vi "Export - Main.vi"(8 "error in (no error)":errorcluster, 11 "Device Item Ref in":T10 format="%.0x") -> (0 "error out":errorcluster, 3 "Import/Export Data":T1 {"Tx Packets"."Tx Packet Data"."Endianness" items=["big-endian"=0, "little-endian"=2]; "Rx Packets"."Rx Packet Data"."Endianness" items=["big-endian"=0, "little-endian"=2]})   [LabVIEW 2016, in "UDP-Custom-Device System Explorer.lvlib"]
uses:
  UDP-Custom-Device System Explorer.lvlib
  <vilib>/NI Veristand/Custom Device API/Custom Device Item Ref.ctl
  Types/XML - New/ImpExp - Data.ctl
  Types/XML - New/ImpExp - Main Data.ctl
  <vilib>/NI Veristand/Custom Device API/Custom Device Item Info.ctl
  Types/XML - New/ImpExp - Rx Packets Data.ctl
  Types/XML - New/ImpExp - Rx Packet Data.ctl
  Shared/Types/Shared - Channel Data Type.ctl
  Shared/Types/Shared - Buffered.PacketInfo.ctl
  Types/XML - New/ImpExp - Tx Packets Data.ctl
  Types/XML - New/ImpExp - Tx Packet Data.ctl
  Property Accessors/Main Accessors.lvlib
  <vilib>/NI VeriStand/Custom Device API/Custom Device API.lvlib
  Shared/UDP-Custom-Device Shared.lvlib
  <vilib>/NI VeriStand/Custom Device Tools/Custom Device Utility Library/Custom Device Utility Library.lvlib
panel:
  out "Controller Path":string
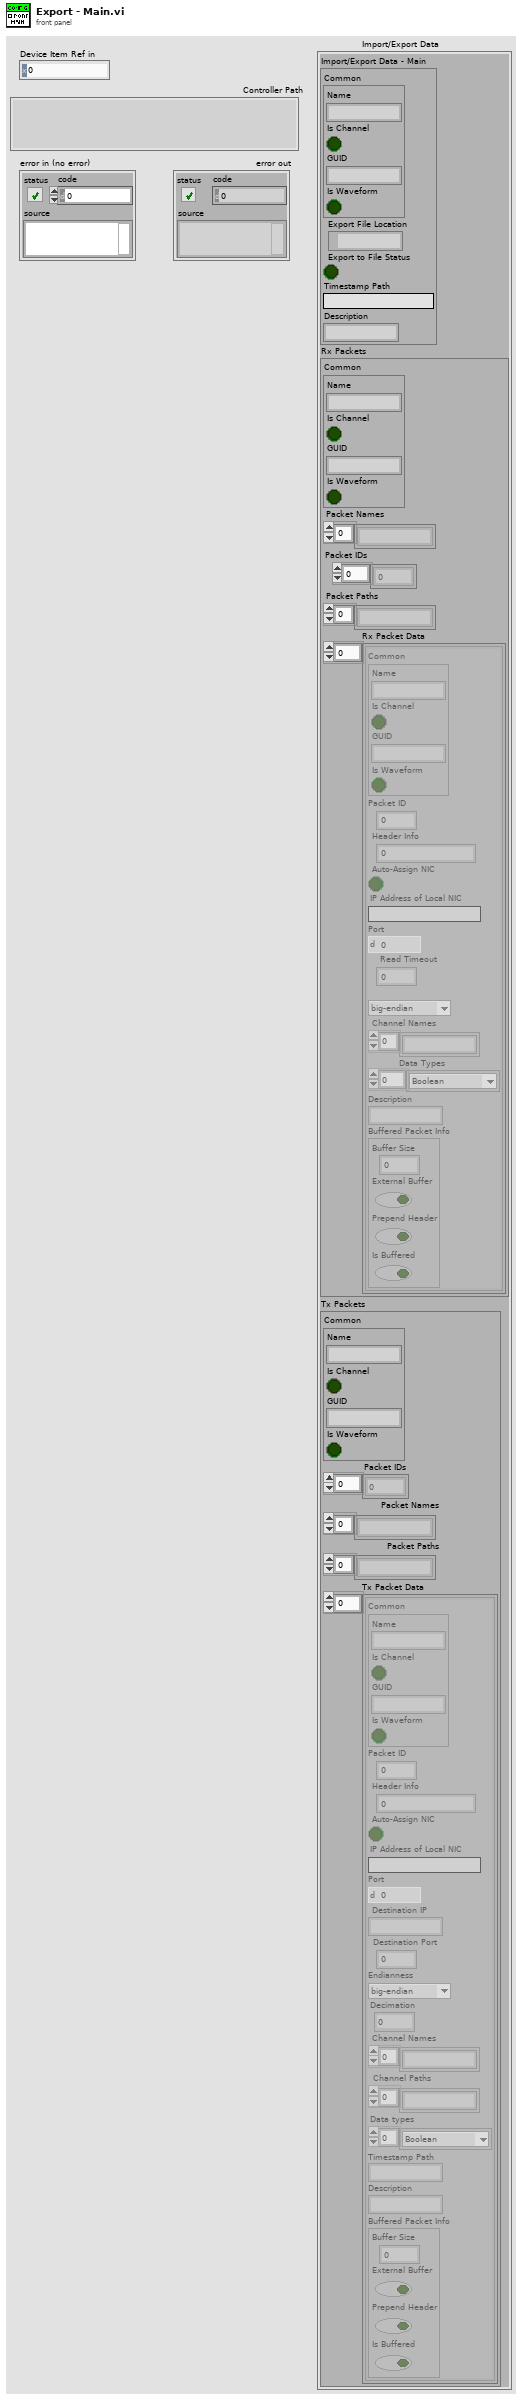
[diagram p1: front panel]
types:
  T1 = typedef "UDP-Custom-Device System Explorer.lvlib/ImpExp - Data.ctl" = cluster{"Import/Export Data - Main":T2, "Rx Packets":T4, "Tx Packets":T8}
  T2 = typedef "UDP-Custom-Device System Explorer.lvlib/ImpExp - Main Data.ctl" = cluster{"Common":T3, "Export File Location":path, "Export to File Status":bool, "Timestamp Path":string, "Description":string}
  T3 = typedef "Custom Device API.lvlib/Custom Device Item Info.ctl" = cluster{"Name":string, "Is Channel":bool, "GUID":string, "Is Waveform":bool}
  T4 = typedef "UDP-Custom-Device System Explorer.lvlib/ImpExp - Rx Packets Data.ctl" = cluster{"Common":T3, "Packet Names":string[], "Packet IDs":i32[], "Packet Paths":string[], "Rx Packet Data":T5[]}
  T5 = typedef "UDP-Custom-Device System Explorer.lvlib/ImpExp - Rx Packet Data.ctl" = cluster{"Common":T3, "Packet ID":i32, "Header Info":u32, "Auto-Assign NIC":bool, "IP Address of Local NIC":string, "Port":u16, "Read Timeout":i32, "Endianness":u16, "Channel Names":string[], "Data Types":T6[], "Description":string, "Buffered Packet Info":T7}
  T6 = typedef "UDP-Custom-Device Shared.lvlib/Shared - Channel Data Type.ctl" = enum16{"Boolean", "Single", "Double", "I8", "I16", "I32", "I64", "U8", "U16", "U32", "U64"}
  T7 = typedef "UDP-Custom-Device Shared.lvlib/Shared - Buffered.PacketInfo.ctl" = cluster{"Buffer Size":i32, "External Buffer":bool, "Prepend Header":bool, "Is Buffered":bool}
  T8 = typedef "UDP-Custom-Device System Explorer.lvlib/ImpExp - Tx Packets Data.ctl" = cluster{"Common":T3, "Packet IDs":i32[], "Packet Names":string[], "Packet Paths":string[], "Tx Packet Data":T9[]}
  T9 = typedef "UDP-Custom-Device System Explorer.lvlib/ImpExp - Tx Packet Data.ctl" = cluster{"Common":T3, "Packet ID":i32, "Header Info":u32, "Auto-Assign NIC":bool, "IP Address of Local NIC":string, "Port":u16, "Destination IP":string, "Destination Port":u16, "Endianness":u16, "Decimation":u16, "Channel Names":string[], "Channel Paths":string[], "Data types":T6[], "Timestamp Path":string, "Description":string, "Buffered Packet Info":T7}
  T10 = typedef "Custom Device API.lvlib/Custom Device Item Ref.ctl" = u64
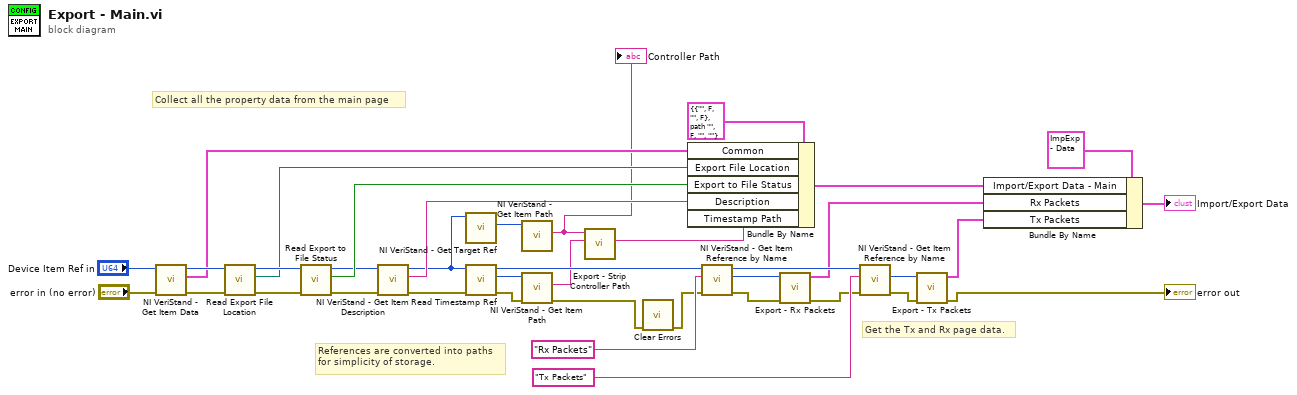
[diagram p0: block diagram]
diagram:
  # "References are converted into paths\nfor simplicity of storage."
  # "Get the Tx and Rx page data."
  # "Collect all the property data from the main page"
  n1 = call <vilib>:"NI VeriStand - Get Item Data.vi"("error in (no error)"="error in (no error)", "Item Ref in"="Device Item Ref in") -> ("error out"=w31:errorcluster, "Item Info"=w28:T3, "Item Ref out"=w33:T10)  [unwired: 6 in, 1 out]
  n2 = call "Read Export File Location.vi"("error in (no error)"=w31, "Node Ptr"=w33) -> ("error out"=w38:errorcluster, "Export File Location"=w27:path, "Node Ptr out"=w37:T10)  [unwired: 7 in]
  n3 = call "Read Export to File Status.vi"("error in (no error)"=w38, "Node Ptr"=w37) -> ("error out"=w9:errorcluster, "Export to File Status"=w26:bool, "Node Ptr out"=w6:T10)  [unwired: 7 in]
  n4 = call <vilib>:"NI VeriStand - Get Item Description.vi"("error in (no error)"=w9, "Item Ref in"=w6) -> ("error out"=w8:errorcluster, "Description"=w5:string, "Item Ref out"=w4:T10)  [unwired: 6 in, 1 out]
  n5 = call <vilib>:"NI VeriStand - Get Target Ref.vi"("Item Ref in"=w4) -> ("Target Ref"=w7:T10)  [unwired: 7 in, 3 out]
  n6 = call "Read Timestamp Ref.vi"("error in (no error)"=w8, "Node Ptr"=w4) -> ("error out"=w35:errorcluster, "Timestamp Ref"=w36:T10, "Node Ptr out"=w24:T10)  [unwired: 7 in]
  n7 = call <vilib>:"NI VeriStand - Get Item Path.vi"("Item Ref in"=w7) -> ("Path"=w1:string)  [unwired: 7 in, 3 out]
  "Controller Path" <- w1
  n8 = call <vilib>:"NI VeriStand - Get Item Path.vi"("error in (no error)"=w35, "Item Ref in"=w36) -> ("error out"=w11:errorcluster, "Path"=w3:string)  [unwired: 6 in, 2 out]
  n9 = call "Export - Strip Controller Path.vi"("Channel Path"=w3, "Controller Path"=w1) -> ("Stripped Path"=w2:string)  [unwired: 8 in, 1 out]
  n10 = call <vilib>:"Clear Errors.vi"("error in (no error)"=w11) -> ("error out"=w10:errorcluster)  [unwired: 5 in, 1 out]
  n11 = Bundle By Name(cluster=T2 {"Common"={"Name"="", "Is Channel"=FALSE, "GUID"="", "Is Waveform"=FALSE}, "Export File Location"=path "", "Export to File Status"=FALSE, "Timestamp Path"="", "Description"=""} ("Import/Export Data - Main"), "Common"=w28, "Export File Location"=w27, "Export to File Status"=w26, "Description"=w5, "Timestamp Path"=w2) -> (w29:T2)
  n12 = call <vilib>:"NI VeriStand - Get Item Reference by Name.vi"("error in (no error)"=w10, "Item Name"="Rx Packets" ("Section Name"), "Parent Ref in"=w24) -> ("error out"=w17:errorcluster, "Item Ref"=w19:T10, "Parent Ref out"=w22:T10)  [unwired: 5 in, 1 out]
  n13 = call "Export - Rx Packets.vi"("error in (no error)"=w17, "Device Item Ref in"=w19) -> ("error out"=w16:errorcluster, "Rx Packets"=w18:T4)  [unwired: 8 in]
  n14 = call <vilib>:"NI VeriStand - Get Item Reference by Name.vi"("error in (no error)"=w16, "Item Name"="Tx Packets" ("Section Name"), "Parent Ref in"=w22) -> ("error out"=w13:errorcluster, "Item Ref"=w15:T10)  [unwired: 5 in, 2 out]
  n15 = call "Export - Tx Packets.vi"("error in (no error)"=w13, "Device Item Ref in"=w15) -> ("error out"=→"error out":errorcluster, "Tx Packets"=w14:T8)  [unwired: 8 in]
  n16 = Bundle By Name(cluster=T1 {"Import/Export Data - Main"={"Common"={"Name"="", "Is Channel"=FALSE, "GUID"="", "Is Waveform"=FALSE}, "Export File Location"=path "", "Export to File Status"=FALSE, "Timestamp Path"="", "Description"=""}, "Rx Packets"={"Common"={"Name"="", "Is Channel"=FALSE, "GUID"="", "Is Waveform"=FALSE}, "Packet Names"=[], "Packet IDs"=[], "Packet Paths"=[], "Rx Packet Data"=[]}, "Tx Packets"={"Common"={"Name"="", "Is Channel"=FALSE, "GUID"="", "Is Waveform"=FALSE}, "Packet IDs"=[], "Packet Names"=[], "Packet Paths"=[], "Tx Packet Data"=[]}} ("Import/Export Data"), "Import/Export Data - Main"=w29, "Rx Packets"=w18, "Tx Packets"=w14) -> (→"Import/Export Data":T1)
